vi "Main.vi"(1 "bot array":dbl[](array[numeric])) -> (0 "XY array":cluster{dbl[], dbl[]}[](array[cluster]))   [LabVIEW 2013]
panel:
  out "size y history":i32
  out "size y wall history":i32
  out "x Wall history":dbl[](array[numeric])
  out "y Wall history":dbl[](array[numeric])
  out "Heading history":dbl[](array[numeric])
  out "X history":dbl[](array[numeric])
  out "Y history":dbl[](array[numeric])
  out "Encoder Right":dbl[](array[numeric])
  out "Encoder Left":dbl[](array[numeric])
  out "IR Front":dbl[](array[numeric])
  out "IR Right":dbl[](array[numeric])
  # "IR Right\n\nIR Front\n\nEncoder left\n\nEncoder righ"
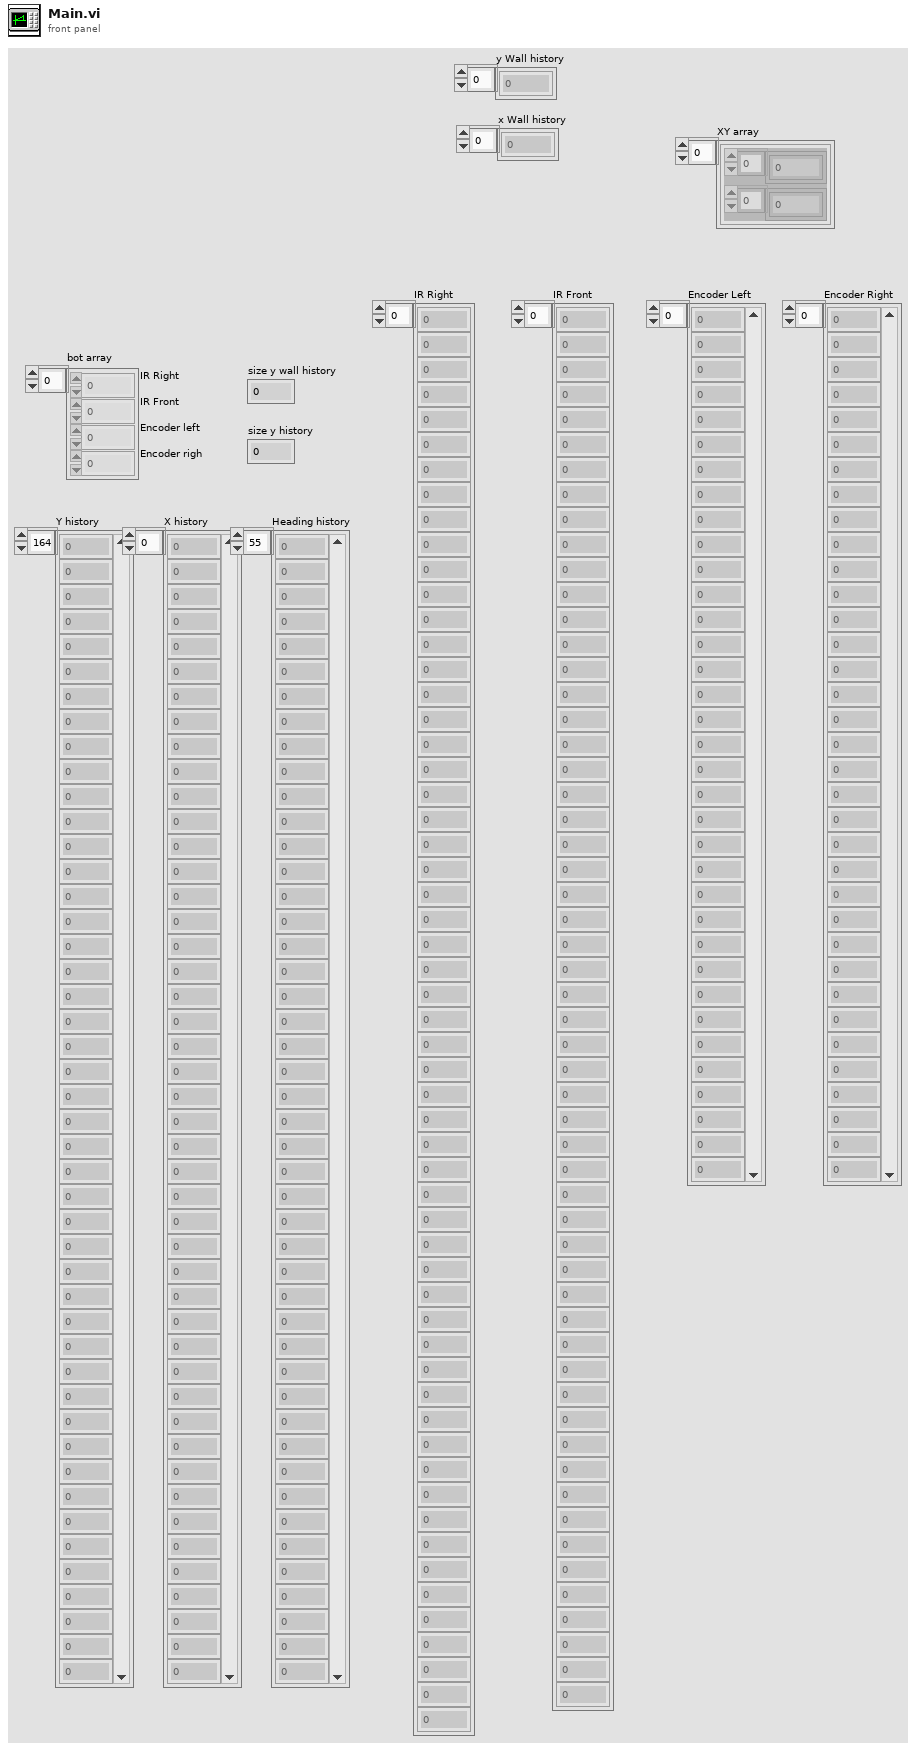
[diagram p1: front panel]
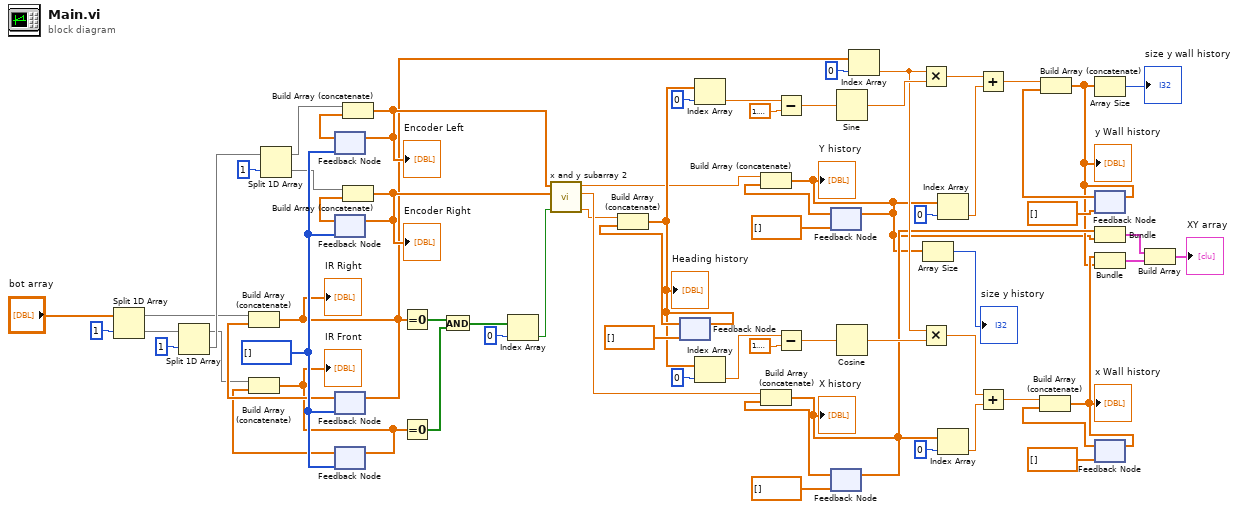
[diagram p0: block diagram]
diagram:
  w67 = i32[] []
  n1 = Split 1D Array(array="bot array", index=1) -> (first subarray=w55:dbl[], second subarray=w62:dbl[])
  n2 = Split 1D Array(array=w62, index=1) -> (first subarray=w52:dbl[], second subarray=w63:dbl[])
  n3 = Split 1D Array(array=w63, index=1) -> (first subarray=w51:dbl[], second subarray=w48:dbl[])
  n4 = feedback #1(w67) -> (w50:dbl[])
  n5 = feedback #2(w67) -> (w49:dbl[])
  n6 = feedback #3(w67) -> (w54:dbl[])
  n7 = Build Array (concatenate)(w55, w54) -> (w6:dbl[])
  "IR Right" <- w6
  n8 = feedback-in #3(w6) -> ()
  n9 = feedback #4(w67) -> (w53:dbl[])
  n10 = Build Array (concatenate)(w52, w53) -> (w5:dbl[])
  "IR Front" <- w5
  n11 = feedback-in #4(w5) -> ()
  n12 = Build Array (concatenate)(w51, w50) -> (w17:dbl[])
  "Encoder Left" <- w17
  n13 = feedback-in #1(w17) -> ()
  n14 = Build Array (concatenate)(w48, w49) -> (w8:dbl[])
  "Encoder Right" <- w8
  n15 = feedback-in #2(w8) -> ()
  n16 = Equal To 0?(x=w6) -> (x = 0?=w4:bool[])
  n17 = Equal To 0?(x=w5) -> (x = 0?=w7:bool[])
  n18 = And(x=w4, y=w7) -> (x .and. y?=w3:bool[])
  n19 = Index Array(array=w3, index=0) -> (element=w1:bool)
  n20 = call "x and y subarray 2.vi"("Turn on itself"=w1, "Encoder  Right"=w8, "Encoder Left"=w17) -> ("Heading"=w14:dbl, "x"=w16:dbl, "y"=w15:dbl)  [unwired: 6 in]
  n21 = feedback #5(dbl[] []) -> (w57:dbl[])
  n22 = Build Array (concatenate)(w14, w57) -> (w32:dbl[])
  "Heading history" <- w32
  n23 = feedback-in #5(w32) -> ()
  n24 = Index Array(array=w32, index=0) -> (element=w44:dbl)
  n25 = Index Array(array=w32, index=0) -> (element=w36:dbl)
  n26 = Subtract(x=w44, y=1.5707963267948966) -> (x-y=w43:dbl)
  n27 = Subtract(x=w36, y=1.5707963267948966) -> (x-y=w37:dbl)
  n28 = feedback #6(dbl[] []) -> (w61:dbl[])
  n29 = Build Array (concatenate)(w15, w61) -> (w9:dbl[])
  "Y history" <- w9
  n30 = feedback-in #6(w9) -> ()
  n31 = feedback #7(dbl[] []) -> (w58:dbl[])
  n32 = Build Array (concatenate)(w16, w58) -> (w18:dbl[])
  "X history" <- w18
  n33 = feedback-in #7(w18) -> ()
  n34 = Sine(x=w43) -> (sin(x)=w47:dbl)
  n35 = Cosine(x=w37) -> (cos(x)=w34:dbl)
  n36 = Index Array(array=w6, index=0) -> (element=w26:dbl)
  n37 = Multiply(x=w26, y=w47) -> (x*y=w28:dbl)
  n38 = Multiply(x=w26, y=w34) -> (x*y=w22:dbl)
  n39 = Array Size(array=w9) -> (size(s)=→"size y history":i32)
  n40 = Index Array(array=w9, index=0) -> (element=w24:dbl)
  n41 = Index Array(array=w18, index=0) -> (element=w21:dbl)
  n42 = Add(x=w28, y=w24) -> (x+y=w27:dbl)
  n43 = Add(x=w22, y=w21) -> (x+y=w20:dbl)
  n44 = feedback #8(dbl[] []) -> (w41:dbl[])
  n45 = Build Array (concatenate)(w27, w41) -> (w11:dbl[])
  "y Wall history" <- w11
  n46 = Array Size(array=w11) -> (size(s)=→"size y wall history":i32)
  n47 = feedback-in #8(w11) -> ()
  n48 = Bundle(w18, w9) -> (w31:cluster{dbl[], dbl[]})  [unwired: 1 in]
  n49 = feedback #9(dbl[] []) -> (w38:dbl[])
  n50 = Build Array (concatenate)(w20, w38) -> (w19:dbl[])
  "x Wall history" <- w19
  n51 = Bundle(w19, w11) -> (w30:cluster{dbl[], dbl[]})  [unwired: 1 in]
  n52 = feedback-in #9(w19) -> ()
  n53 = Build Array(w31, w30) -> (→"XY array":cluster{dbl[], dbl[]}[])
